vi "new Maze.vi"(8 "error in (no error)":errorcluster) -> (0 "error out":errorcluster, 3 "Maze out":refnum<class "Maze.lvclass">)   [LabVIEW 2016, in "Maze.lvclass"]
uses:
  Maze.lvclass
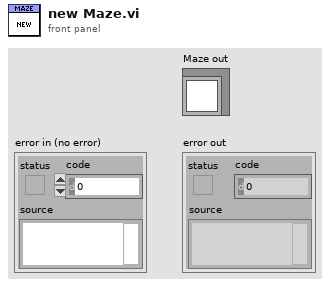
[diagram p1: front panel]
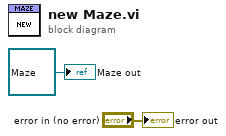
[diagram p0: block diagram]
diagram:
  "error out" <- "error in (no error)"
  "Maze out" <- refnum<class "Maze.lvclass"> refnum ("Maze in")
